vi "LabelDragMultiThearding.vi"() -> ()   [LabVIEW 2012]
uses:
  <vilib>/Utility/miscctls.llb/LVPositionTypeDef.ctl
  <vilib>/Utility/miscctls.llb/LVBoundsTypeDef.ctl
  <vilib>/Utility/miscctls.llb/LVPoint32TypeDef.ctl
panel:
  out "StopState":bool
  out "边界 2":T1 caption="边界"
  out "时间":u32
  out "数值":i32
  out "x-y":T2
  out "位置 2":T3 caption="位置"
  out "坐标":T2 caption="鼠标按下时坐标"
  out "拖动state":bool
  in  "等待时间（毫秒）":u32=100
  in  "停止":bool
  out "二维图片":picture
  out "边界":T1
  out "位置":T3
  out "波形图":dbl[](graph)
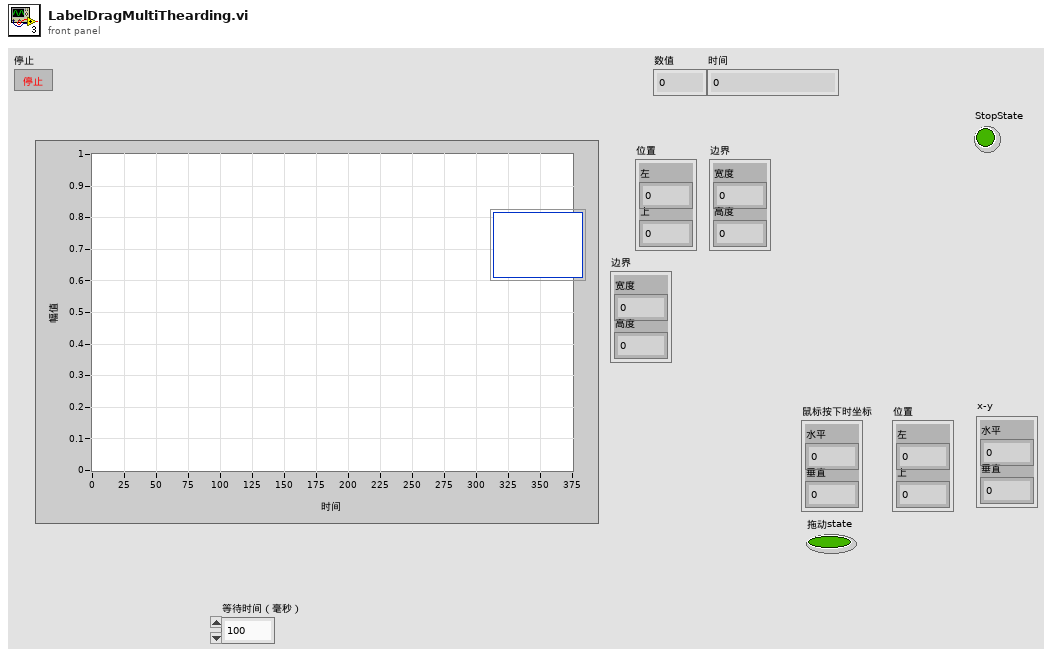
[diagram p1: front panel]
types:
  T1 = typedef "LVBoundsTypeDef.ctl" = cluster{"Width":u32, "Height":u32}
  T2 = typedef "LVPoint32TypeDef.ctl" = cluster{"Horizontal":i32, "Vertical":i32}
  T3 = typedef "LVPositionTypeDef.ctl" = cluster{"Left":i32, "Top":i32}
  T4 = cluster{"plot name":string, "plot color":u32, "fill?(F)":bool}[]
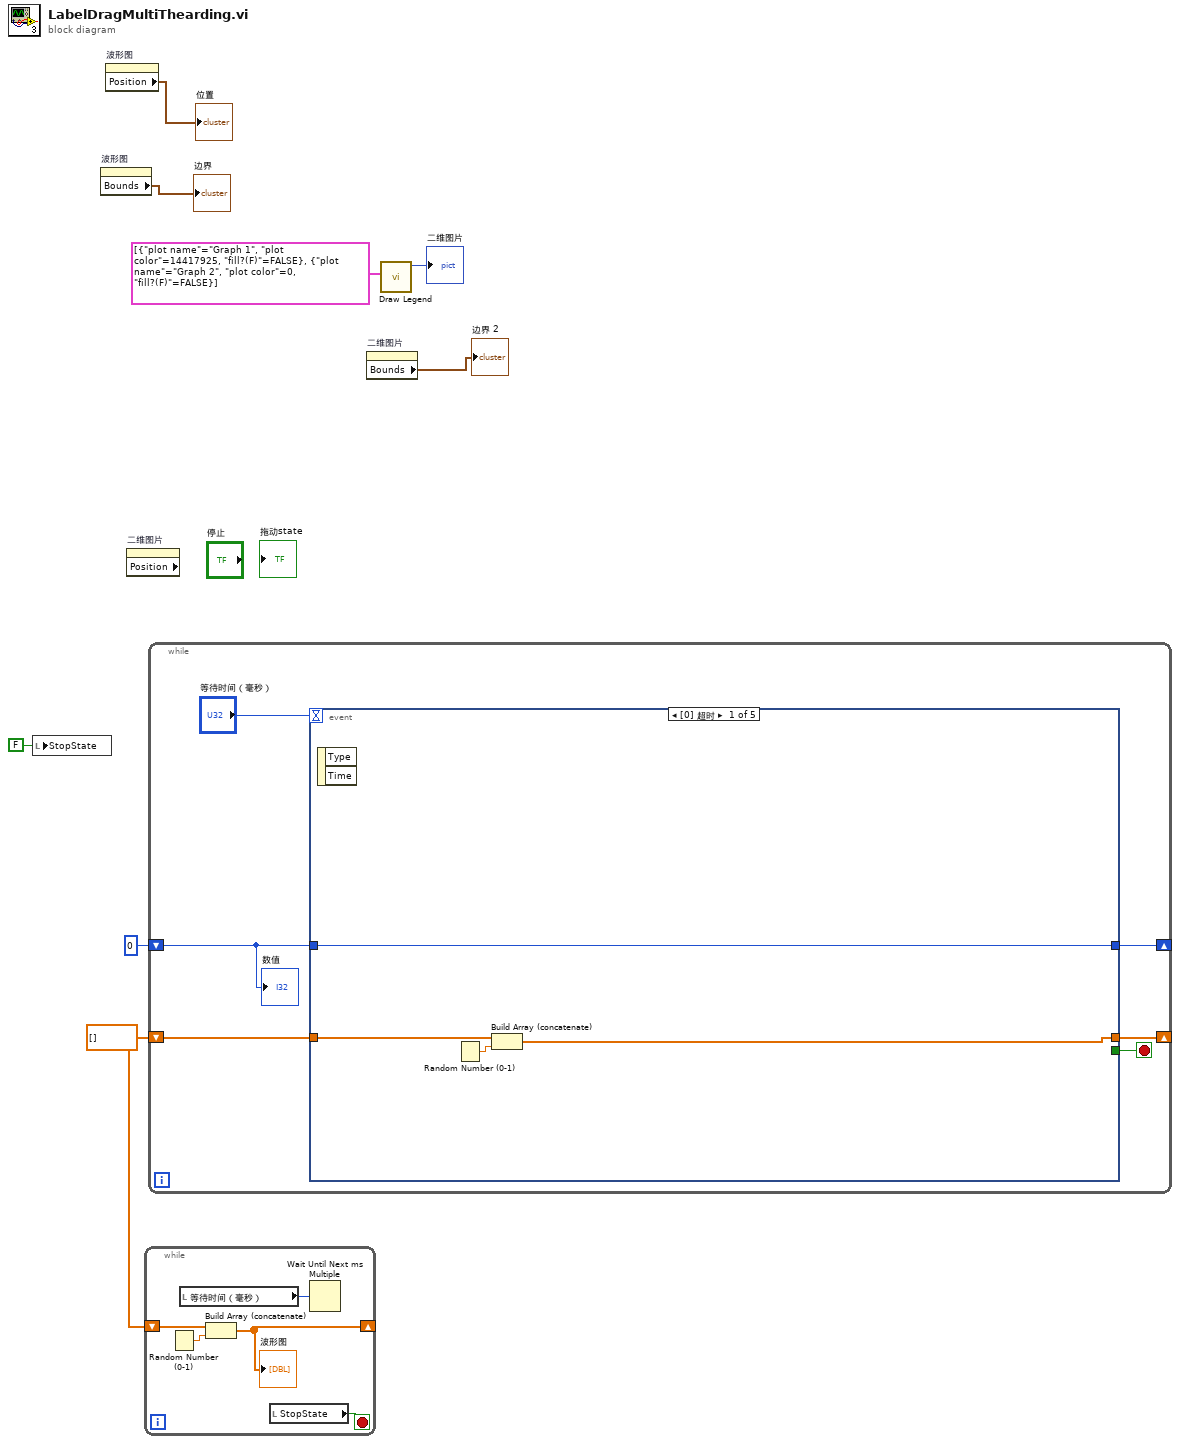
[diagram p0: block diagram]
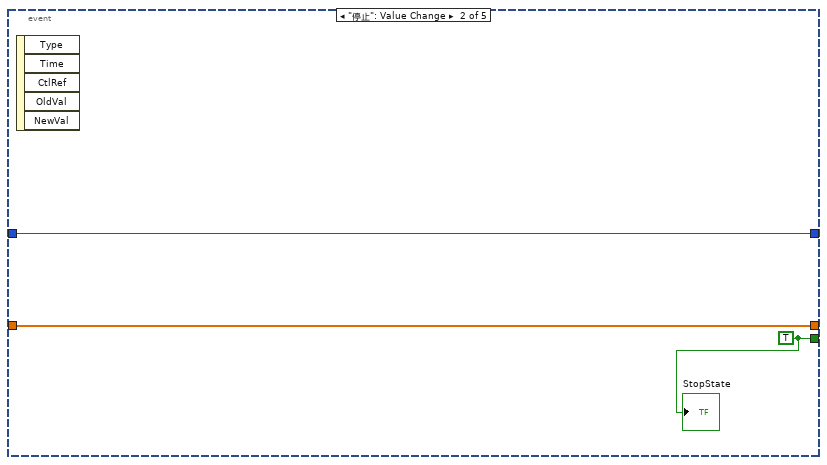
[diagram p2: hidden frame]
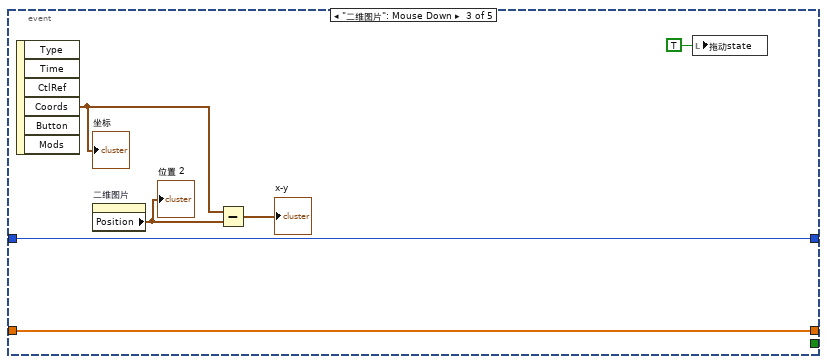
[diagram p3: hidden frame]
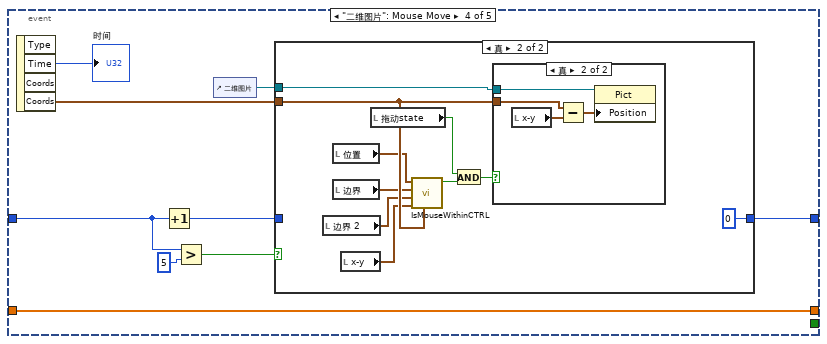
[diagram p4: hidden frame]
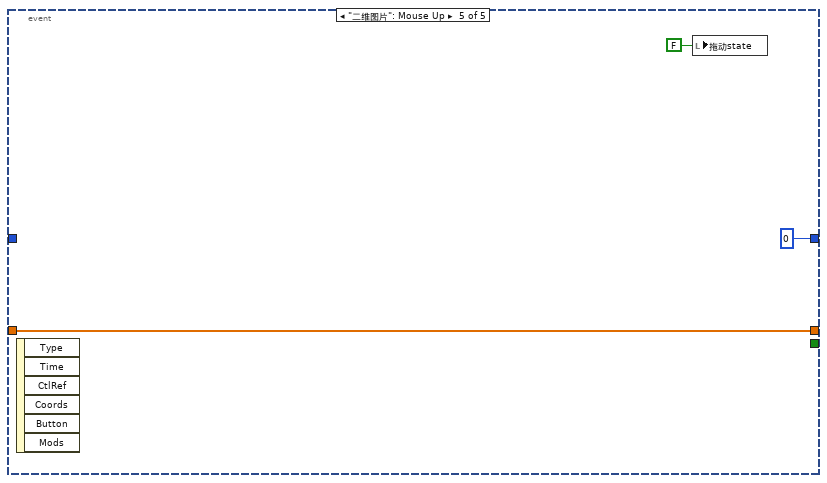
[diagram p7: hidden frame]
diagram:
  w2 = dbl[] []
  n1 = local write "StopState"(FALSE ("StopState")) -> ()
  n2 = property on="波形图" class="WFGraph (严格)"() -> ("Bounds"=→"边界":T1)  [unwired: 2 in, 2 out]
  n3 = property on="波形图" class="WFGraph (严格)"() -> ("Position"=→"位置":T3)  [unwired: 2 in, 2 out]
  n4 = property on="二维图片" class="Pict" props=["Position"]() -> ()  [unwired: 2 in, 3 out]
  n5 = while {
    shift-right: [w10] -> _
    shift-left: w2 -> [w11]
    stop <- w13 stop-if-true
    n6 = Random Number (0-1)() -> (number: 0 to 1=w12:dbl)
    n7 = local read "等待时间（毫秒）"() -> (w9:u32)
    n8 = Build Array (concatenate)(w11, w12) -> (w10:dbl[])
    "波形图" <- w10
    n9 = local read "StopState"() -> (w13:bool)
    n10 = Wait Until Next ms Multiple(millisecond multiple=w9) -> ()  [unwired: 1 out]
  }
  n11 = while {
    shift-right: [w17] -> _
    shift-left: w2 -> [w18]
    shift-right: [w14] -> _
    shift-left: 0 -> [w15]
    stop <- w16 stop-if-true
    n12 = event shown="[0] 超时" {
      selector: _ -> [_ _ _ _ _]
      dyn-events: _ -> [_ _ _ _ _]
      timeout: "等待时间（毫秒）" -> [_ _ _ _ _]
      tunnel: w18 -> [w22 w26 w31 w40 w58]
      tunnel: [w21 w26 w31 w40 w58] -> w17
      tunnel: [_ w24 _ _ _] -> w16
      tunnel: [w20 w25 w27 w38 0] -> w14
      tunnel: w15 -> [w20 w25 w27 w36 _]
      event Timeout {
        n13 = event-data() -> ()  [unwired: 1 in, 2 out]
        n14 = Random Number (0-1)() -> (number: 0 to 1=w23:dbl)
        n15 = Build Array (concatenate)(w22, w23) -> (w21:dbl[])
      }
      event "停止": Value Change {
        w24 = TRUE
        n16 = event-data() -> ()  [unwired: 1 in, 5 out]
        "StopState" <- w24
      }
      event "二维图片": Mouse Down {
        n17 = event-data() -> ("Coords"=w30:T2)  [unwired: 1 in, 5 out]
        "坐标" <- w30
        n18 = property on="二维图片" class="Pict"() -> ("Position"=w29:T3)  [unwired: 2 in, 2 out]
        "位置 2" <- w29
        n19 = Subtract(x=w30, y=w29) -> (x-y=→"x-y":T2)
        n20 = local write "拖动state"(TRUE ("拖动state")) -> ()
      }
      event "二维图片": Mouse Move {
        n21 = event-data() -> ("Time"=→"时间":u32, "Coords"=w41:T2)  [unwired: 1 in, 2 out]
        n22 = Increment(x=w36) -> (x+1=w35:i32)
        n23 = Greater?(x=w36, y=5) -> (0:w39:bool)
        n24 = control-ref of="二维图片"() -> (w34:refnum<vi>)
        n25 = case shown="真" w39 {
          tunnel: w34 -> [_ w52]
          tunnel: w41 -> [_ w50]
          tunnel: [w42 0 ("y")] -> w38
          tunnel: w35 -> [w42 _]
          frame False {
          }
          frame True {
            n26 = local read "边界 2"() -> (w46:T1)
            n27 = local read "位置"() -> (w48:T3)
            n28 = local read "边界"() -> (w47:T1)
            n29 = local read "x-y"() -> (w49:T2)
            n30 = local read "拖动state"() -> (w45:bool)
            n31 = call "IsMouseWithinCTRL.vi"("鼠标坐标"=w50, "x-y"=w49, "图例边界"=w46, "控件边界"=w47, "控件位置"=w48) -> ("IsMouseWithin"=w44:bool)  [unwired: 6 in]
            n32 = And(x=w45, y=w44) -> (x .and. y?=w43:bool)
            n33 = case shown="真" w43 {
              tunnel: w52 -> [_ w56]
              tunnel: w50 -> [_ w55]
              frame False {
              }
              frame True {
                n34 = local read "x-y"() -> (w54:T2)
                n35 = Subtract(x=w55, y=w54) -> (x-y=w53:T2)
                n36 = property class="Pict"(reference=w56, "Position"=w53) -> ()  [unwired: 1 in, 2 out]
              }
            }
          }
        }
      }
      event "二维图片": Mouse Up {
        n37 = event-data() -> ()  [unwired: 1 in, 6 out]
        n38 = local write "拖动state"(FALSE ("拖动state")) -> ()
      }
    }
    "数值" <- w15
  }
  n39 = property on="二维图片" class="Pict"() -> ("Bounds"=→"边界 2":T1)  [unwired: 2 in, 2 out]
  n40 = call <vilib>:"Draw Legend.vi"("plot info"=T4 [{"plot name"="Graph 1", "plot color"=14417925, "fill?(F)"=FALSE}, {"plot name"="Graph 2", "plot color"=0, "fill?(F)"=FALSE}]) -> ("new picture"=→"二维图片":picture)  [unwired: 10 in]
